vi "Representacion.vi"() -> ()   [LabVIEW 2020]
panel:
  out "Meter":dbl(knob) scale=0.0..10.0
  in  "Control1":dbl(slide) scale=0.0..10.0
  # "Representacion de Datos"
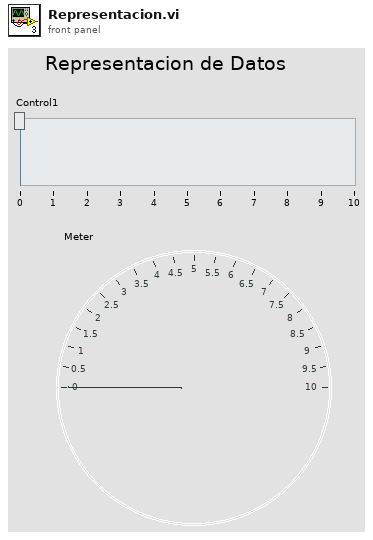
[diagram p1: front panel]
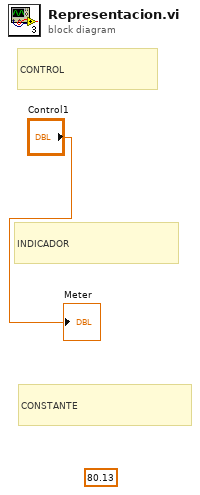
[diagram p0: block diagram]
diagram:
  (unwired) 80.13
  # "CONSTANTE"
  # "INDICADOR"
  # "CONTROL"
  "Meter" <- "Control1"
